vi "RepositionErrorTerminalsVertically.vi"(6 "Error terminals":T1, 8 "error in (no error)":errorcluster, 9 "Item to enclose in case structure":refnum<vi>[](array[refnum]), 11 "VI in":refnum<vi>) -> (0 "error out":errorcluster, 1 "Item to enclose in case structure (dup)":refnum<vi>[](array[refnum]), 3 "VI out (dup)":refnum<vi>)   [LabVIEW 2017, in "ErrorStructureDrawer.lvlib"]
doc: "Selects and moves the specified error control and indicator, in order to move them below the specified items (the ones which will end up in the new case structure)."
uses:
  ErrorStructureDrawer.lvlib
  Controls/ErrorTerminals.ctl
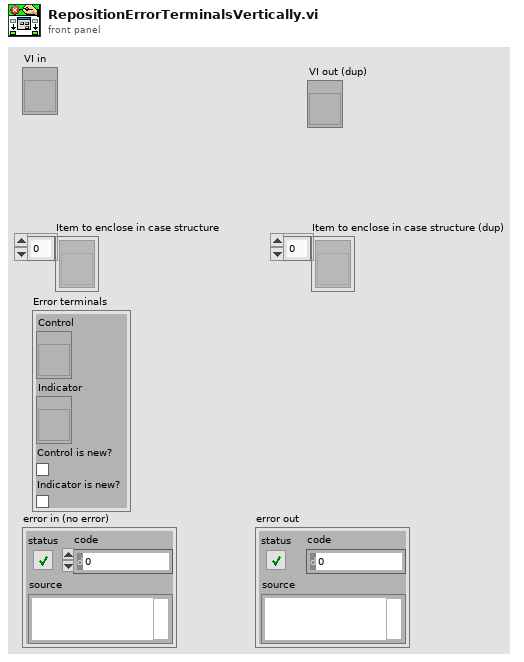
[diagram p1: front panel]
types:
  T1 = typedef "ErrorStructureDrawer.lvlib/ErrorTerminals.ctl" = cluster{"Control":refnum<vi>, "Indicator":refnum<vi>, "Control is new?":bool, "Indicator is new?":bool}
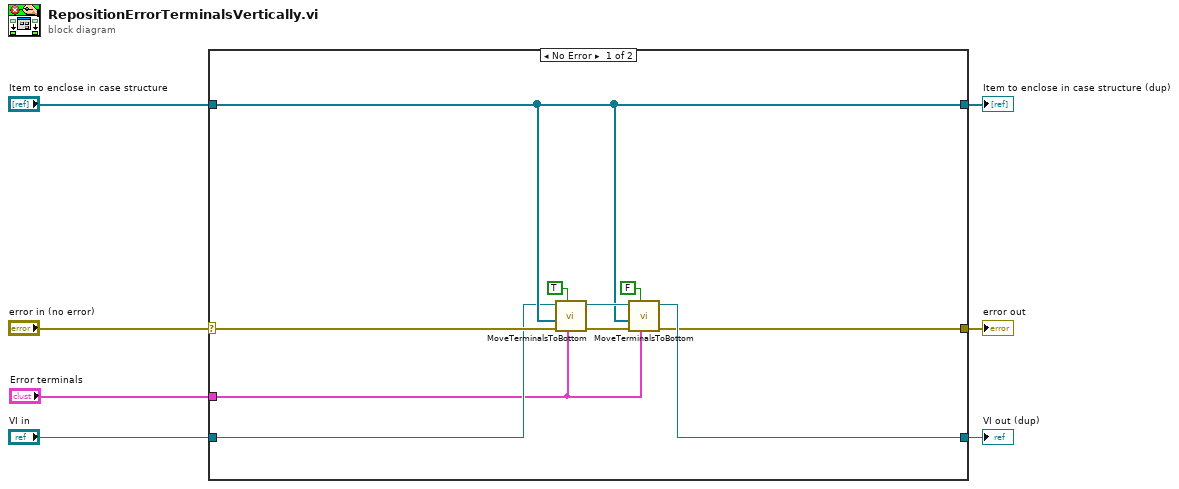
[diagram p0: block diagram]
diagram:
  n1 = case shown="No Error" "error in (no error)" {
    selector: "error in (no error)" -> [w12 w19]
    tunnel: "VI in" -> [w11 w18]
    tunnel: "Item to enclose in case structure" -> [w15 w20]
    tunnel: [w8 w19] -> w5
    tunnel: [w15 w20] -> w4
    tunnel: [w10 w18] -> w2
    tunnel: "Error terminals" -> [w9 _]
    frame No Error {
      n2 = call "MoveTerminalsToBottom.vi"("Error terminals"=w9, "Controls [t] / indicators [f]"=TRUE, "error in (no error)"=w12, "Case structure contents to move away from"=w15, "VI in"=w11) -> ("error out"=w14:errorcluster, "VI ref (dup)"=w16:refnum<vi>)  [unwired: 5 in]
      n3 = call "MoveTerminalsToBottom.vi"("Error terminals"=w9, "Controls [t] / indicators [f]"=FALSE, "error in (no error)"=w14, "Case structure contents to move away from"=w15, "VI in"=w16) -> ("error out"=w8:errorcluster, "VI ref (dup)"=w10:refnum<vi>)  [unwired: 5 in]
    }
    frame Error {
    }
  }
  "error out" <- w5
  "VI out (dup)" <- w2
  "Item to enclose in case structure (dup)" <- w4
